vi "Pre Launch Init.vi"(11 "Algorithm in":refnum<class "Algorithm.lvclass">) -> (0 "error out":errorcluster, 3 "Algorithm out":refnum<class "Algorithm.lvclass">)   [LabVIEW 2019, in "Algorithm.lvclass"]
doc: "(<B>Filename</B>: Actor Framework.lvlib:Actor.lvclass:Pre Launch Init.vi)\n\nDefines behavior that occurs after the Launch Actor method is invoked but before the actor's Actor Core method begins running.\n\nThe Pre Launch Init method is guaranteed to finish before the Launch Actor method returns to its caller and before the actor itself receives any messages. Any references that the Pre Launch Init method obtains are guaranteed to have the same lifetime as the actor itself. Any errors that the Pre Launch Init method returns will abort the launch.\n\nBy default, this method does nothing. A descendant class may override it to define behavior."
uses:
  Algorithm.lvclass
  <vilib>/ActorFramework/Actor/Actor.lvclass
  <vilib>/vision/Image Controls.llb/IMAQ Image.ctl
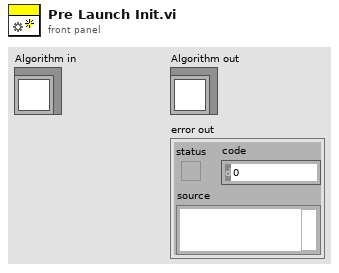
[diagram p1: front panel]
types:
  T1 = typedef "IMAQ Image.ctl" = refnum<image>
  T2 = cluster{"Totalcount":u64, "Reelcount":u64, "PartName":string}
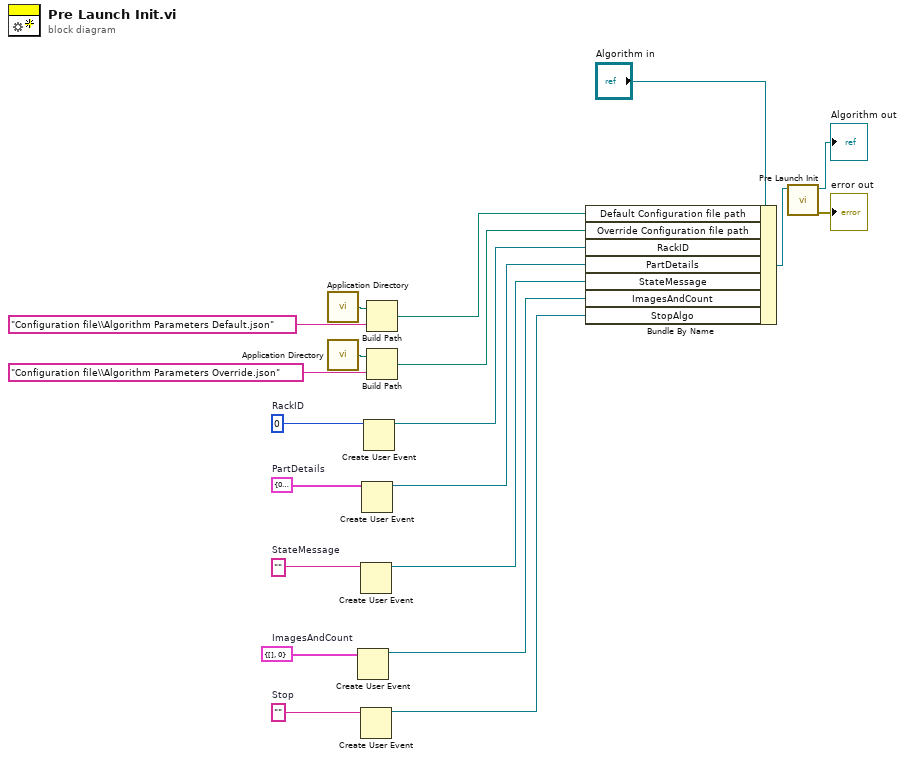
[diagram p0: block diagram]
diagram:
  w2 = ""  # Stop
  w7 = cluster{"Image Array":T1[], "ImageCount":u64} {"Image Array"=[], "ImageCount"=0}  # ImagesAndCount
  w8 = ""  # StateMessage
  w9 = T2 {"Totalcount"=0, "Reelcount"=0, "PartName"=""}  # PartDetails
  w10 = u8 0  # RackID
  n1 = call <vilib>:"Application Directory.vi"() -> ("Application Directory"=w16:path)
  n2 = call <vilib>:"Application Directory.vi"() -> ("Application Directory"=w12:path)
  n3 = Create User Event(user event datatype=w7) -> (user event=w3:refnum<user-event>)  [unwired: 1 in, 1 out]
  n4 = Create User Event(user event datatype=w8) -> (user event=w4:refnum<user-event>)  [unwired: 1 in, 1 out]
  n5 = Create User Event(user event datatype=w2) -> (user event=w1:refnum<user-event>)  [unwired: 1 in, 1 out]
  n6 = Create User Event(user event datatype=w9) -> (user event=w5:refnum<user-event>)  [unwired: 1 in, 1 out]
  n7 = Create User Event(user event datatype=w10) -> (user event=w6:refnum<user-event>)  [unwired: 1 in, 1 out]
  n8 = Build Path(base path=w16, name or relative path="Configuration file\\Algorithm Parameters Default.json") -> (appended path=w14:path)
  n9 = Build Path(base path=w12, name or relative path="Configuration file\\Algorithm Parameters Override.json") -> (appended path=w11:path)
  n10 = Bundle By Name(cluster="Algorithm in", "Default Configuration file path"=w14, "Override Configuration file path"=w11, "RackID"=w6, "PartDetails"=w5, "StateMessage"=w4, "ImagesAndCount"=w3, "StopAlgo"=w1) -> (w18:refnum<class "Algorithm.lvclass">)
  n11 = call-parent "Pre Launch Init.vi"("Actor in"=w18) -> ("error out"=→"error out":errorcluster, "Actor out"=→"Algorithm out":refnum<class "Algorithm.lvclass">)  [unwired: 9 in]
